vi "display.vi"(8 "error in (no error)":errorcluster, 9 "PD  Display":refnum<vi>, 10 "Stop Flag Reference":refnum<vi>, 11 "Photodiode in":refnum<class "Photodiode.lvclass">) -> (0 "error out":errorcluster, 1 "ScanImage Frame Syn":waveform(dbl)(graph), 2 "Photodiode":waveform(dbl)(graph), 3 "Photodiode out":refnum<class "Photodiode.lvclass">)   [LabVIEW 2014, in "Photodiode.lvclass"]
uses:
  Photodiode.lvclass
  Photodiode.lvclass/Photodiode.ctl
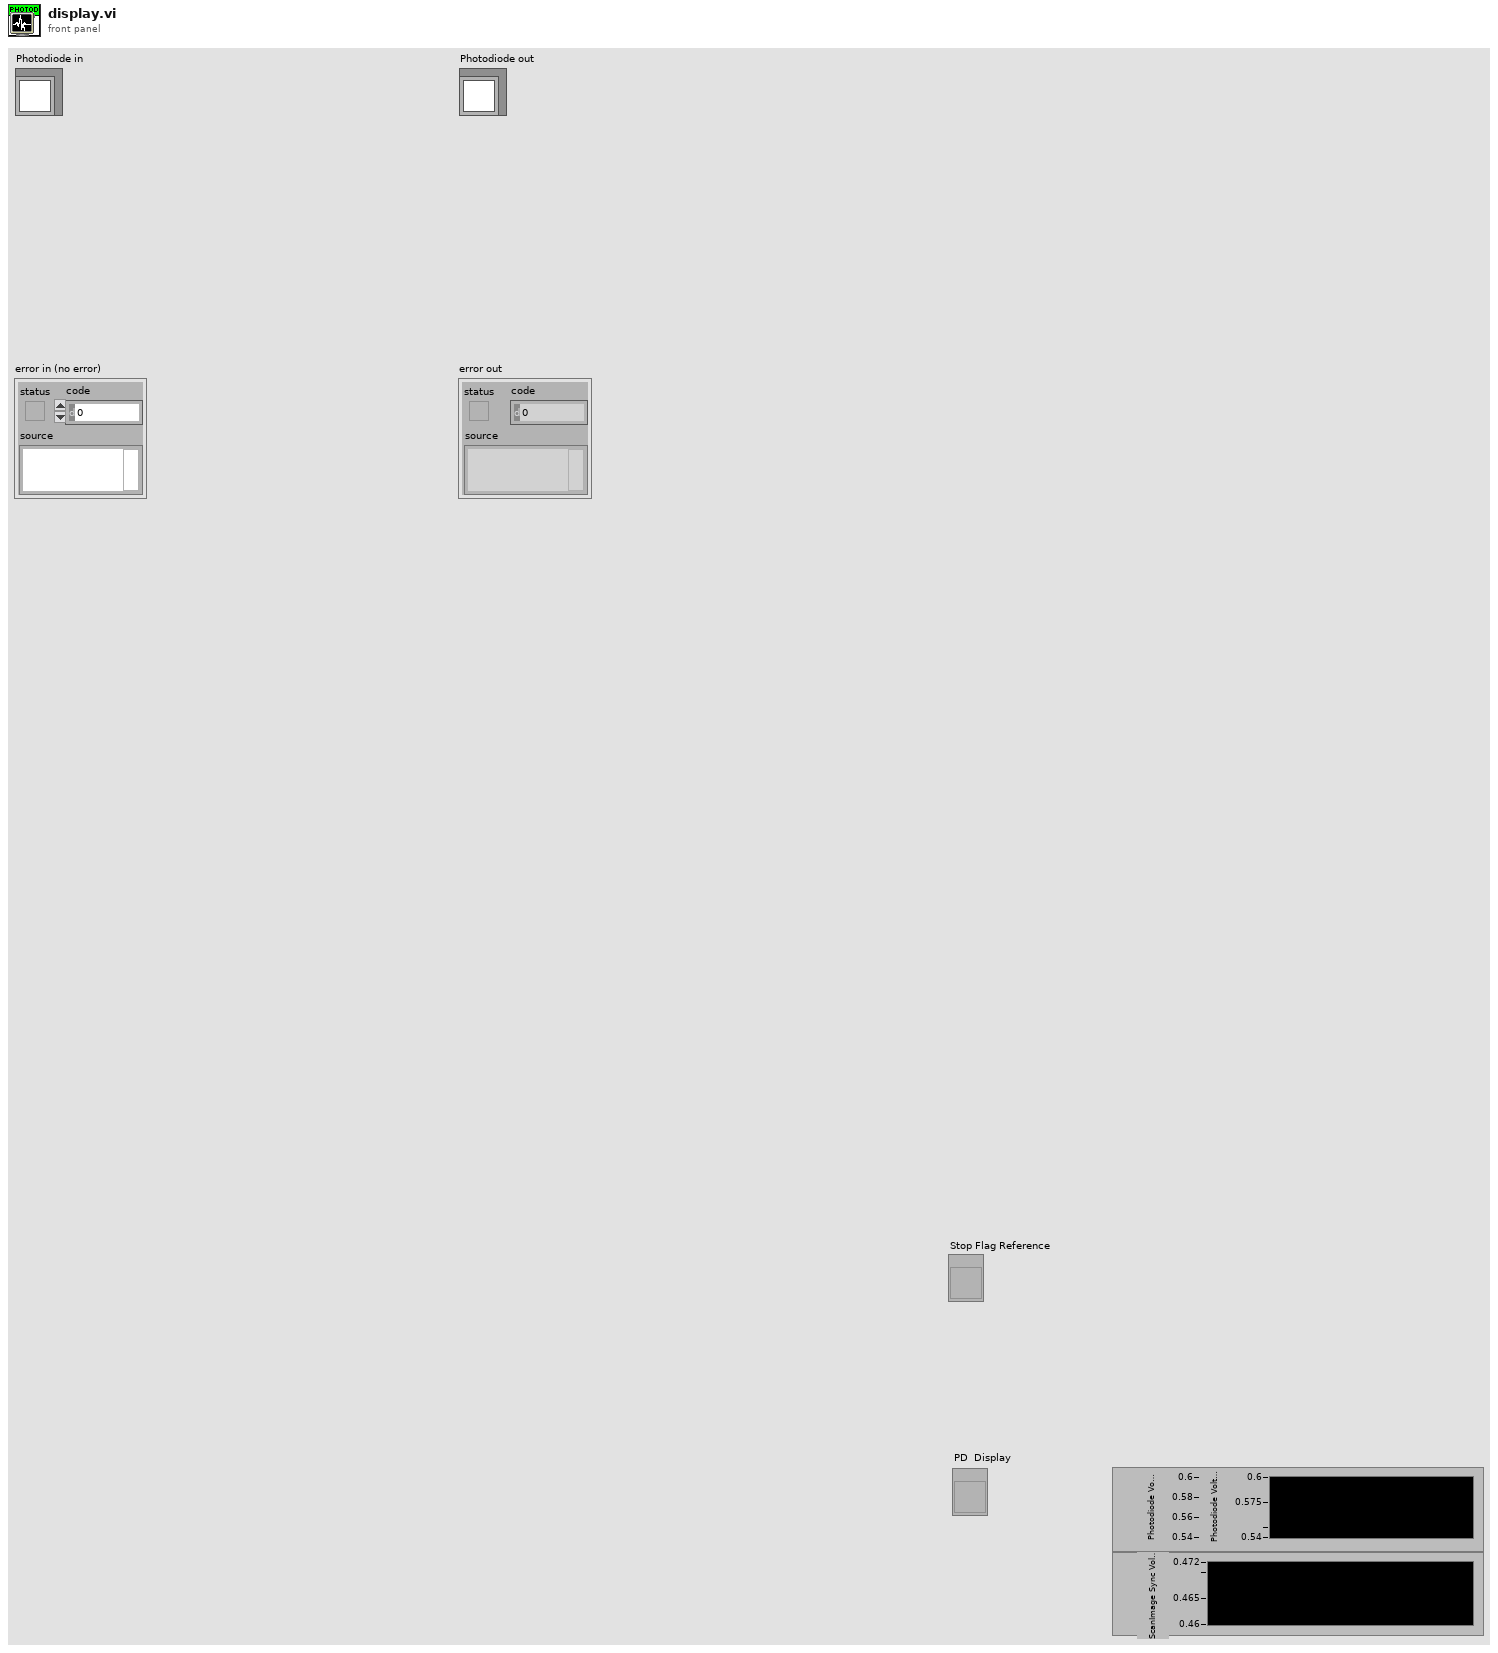
[diagram p1: front panel]
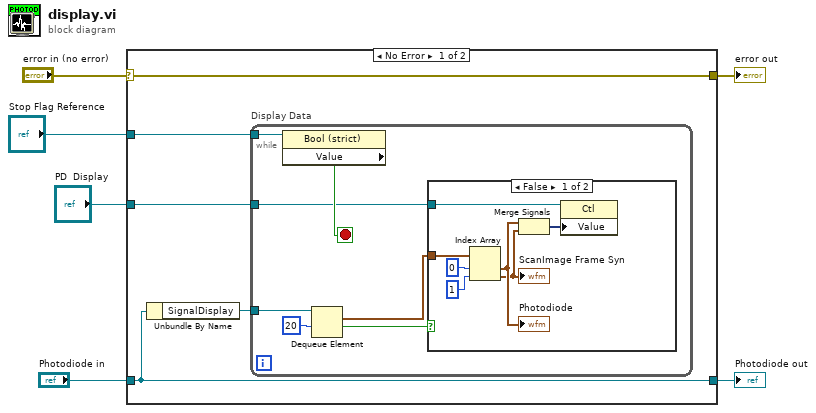
[diagram p0: block diagram]
diagram:
  n1 = case shown="No Error" "error in (no error)" {
    selector: "error in (no error)" -> [w11 w27]
    tunnel: [w11 w27] -> w5
    tunnel: [w9 w26] -> w3
    tunnel: "Photodiode in" -> [w9 w26]
    tunnel: "Stop Flag Reference" -> [w10 _]
    tunnel: "PD  Display" -> [w7 _]
    frame No Error {
      n2 = Unbundle By Name(w9) -> ("SignalDisplay"=w8:refnum<queue>)
      n3 = while "Display Data" {
        tunnel: w8 -> [w16]
        tunnel: w10 -> [w13]
        tunnel: w7 -> [w12]
        stop <- w18 stop-if-true
        n4 = property class="Bool (strict)"(reference=w13) -> ("Value"=w18:bool)  [unwired: 1 in, 2 out]
        n5 = Dequeue Element(queue=w16, timeout in ms (-1)=20) -> (element=w14:waveform(dbl)[], timed out?=w15:bool)  [unwired: 1 in, 2 out]
        n6 = case shown="False" w15 {
          tunnel: w14 -> [w25 _]
          tunnel: w12 -> [w22 _]
          frame False {
            n7 = Index Array(array=w25, index #1=0 ("index"), index #2=1 ("index")) -> (element #1=w21:waveform(dbl), element #2=w20:waveform(dbl))
            "Photodiode" <- w21
            "ScanImage Frame Syn" <- w20
            n8 = Merge Signals(w21, w20) -> (w19:dynamicdata)
            n9 = property class="Ctl"(reference=w22, "Value"=w19) -> ()  [unwired: 1 in, 2 out]
          }
          frame True {
          }
        }
      }
    }
    frame Error {
    }
  }
  "error out" <- w5
  "Photodiode out" <- w3
